vi "ParseSetLogDirectory.vi"(8 "error in (no error)":errorcluster, 11 "message body":variant) -> (0 "error out":errorcluster, 3 "tracepoint directories":T1)   [LabVIEW 2017, in "TraceLogger.lvlib"]
uses:
  <vilib>/addons/TraceLogger/TraceLogger.lvlib
  <vilib>/addons/TraceLogger/controls/TracpointDirectories.ctl
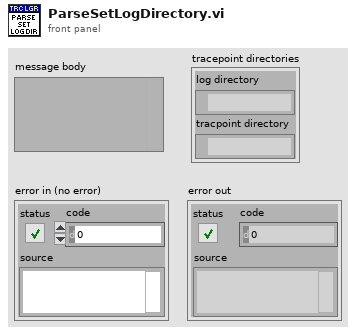
[diagram p1: front panel]
types:
  T1 = typedef "TracpointDirectories.ctl" = cluster{"log directory":path, "tracpoint directory":path}
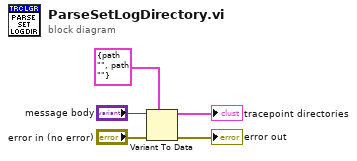
[diagram p0: block diagram]
diagram:
  n1 = Variant To Data(error in="error in (no error)", type=T1 {"log directory"=path "", "tracpoint directory"=path ""} ("tracpoint directories"), Variant="message body") -> (data=→"tracepoint directories":T1, error out=→"error out":errorcluster)
